vi "ReleaseStateQueue.vi"(8 "error in":errorcluster, 11 "QueueIn":variant) -> (0 "error out":errorcluster)   [LabVIEW 2013]
uses:
  Ctl/States.ctl
panel:
  in  "queue out":refnum<queue>
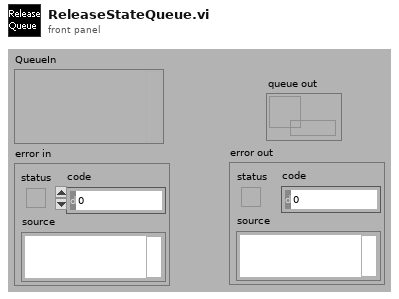
[diagram p1: front panel]
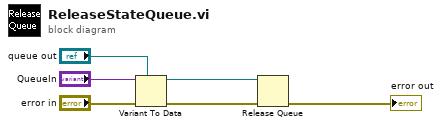
[diagram p0: block diagram]
diagram:
  n1 = Variant To Data(error in="error in", type="queue out", Variant="QueueIn") -> (data=w4:refnum<queue>, error out=w1:errorcluster)
  n2 = Release Queue(queue=w4, error in (no error)=w1) -> (error out=→"error out":errorcluster)  [unwired: 3 out]
